vi "accelero_Sub1.vi"(8 "error in (no error)":errorcluster, 11 "Z-Axis":dbl) -> (0 "error out":errorcluster, 3 "Numeric":dbl)   [LabVIEW 2019]
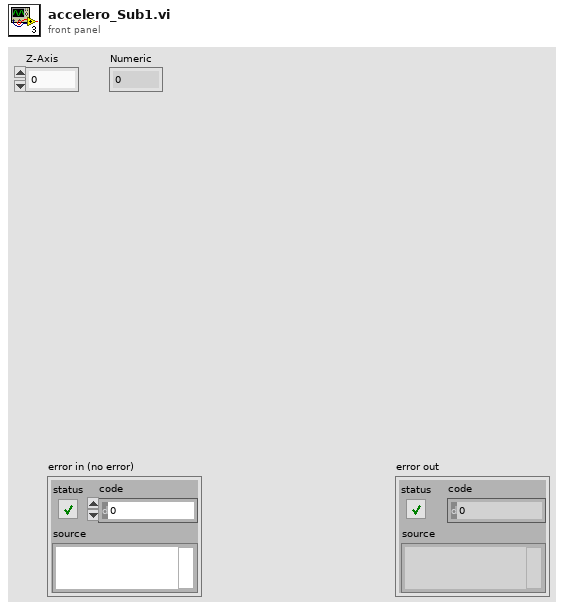
[diagram p1: front panel]
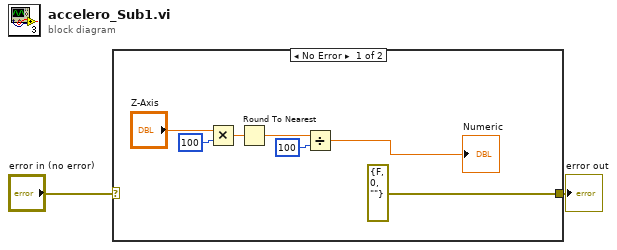
[diagram p0: block diagram]
diagram:
  n1 = case shown="No Error" "error in (no error)" {
    selector: "error in (no error)" -> [_ w10]
    tunnel: [errorcluster {"status"=FALSE, "code"=0, "source"=""} ("error IO") w10] -> w1
    frame No Error {
      n2 = Multiply(x="Z-Axis", y=100) -> (x*y=w8:dbl)
      n3 = Round To Nearest(number=w8) -> (nearest integer value=w7:dbl)
      n4 = Divide(x=w7, y=100) -> (x/y=→"Numeric":dbl)
    }
    frame Error {
    }
  }
  "error out" <- w1
